vi "S7 Write.vi"(6 "Data Type":enum16{"I", "Q", "M", "D", "Count", "Timer"}(ring), 7 "DB block":u16, 8 "Error In":errorcluster, 9 "Write Byte":u8[](array[numeric]), 10 "Start Address":u16, 11 "TCP In":refnum<k5>) -> (0 "Error out":errorcluster caption="Error Out", 3 "TCP Out":refnum<k5>)   [LabVIEW 2020]
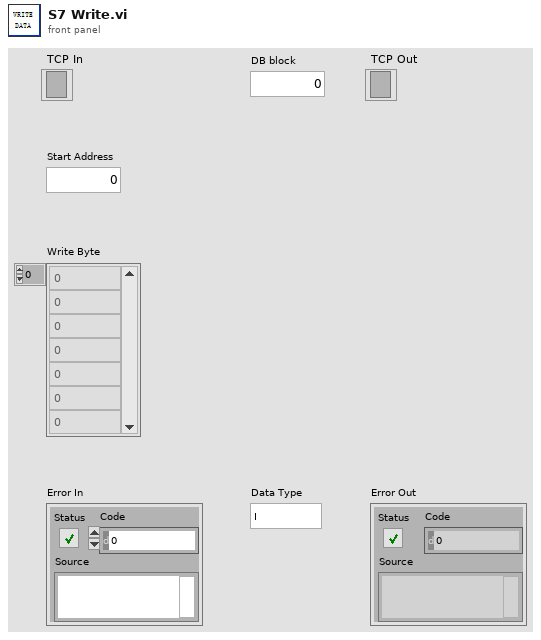
[diagram p1: front panel]
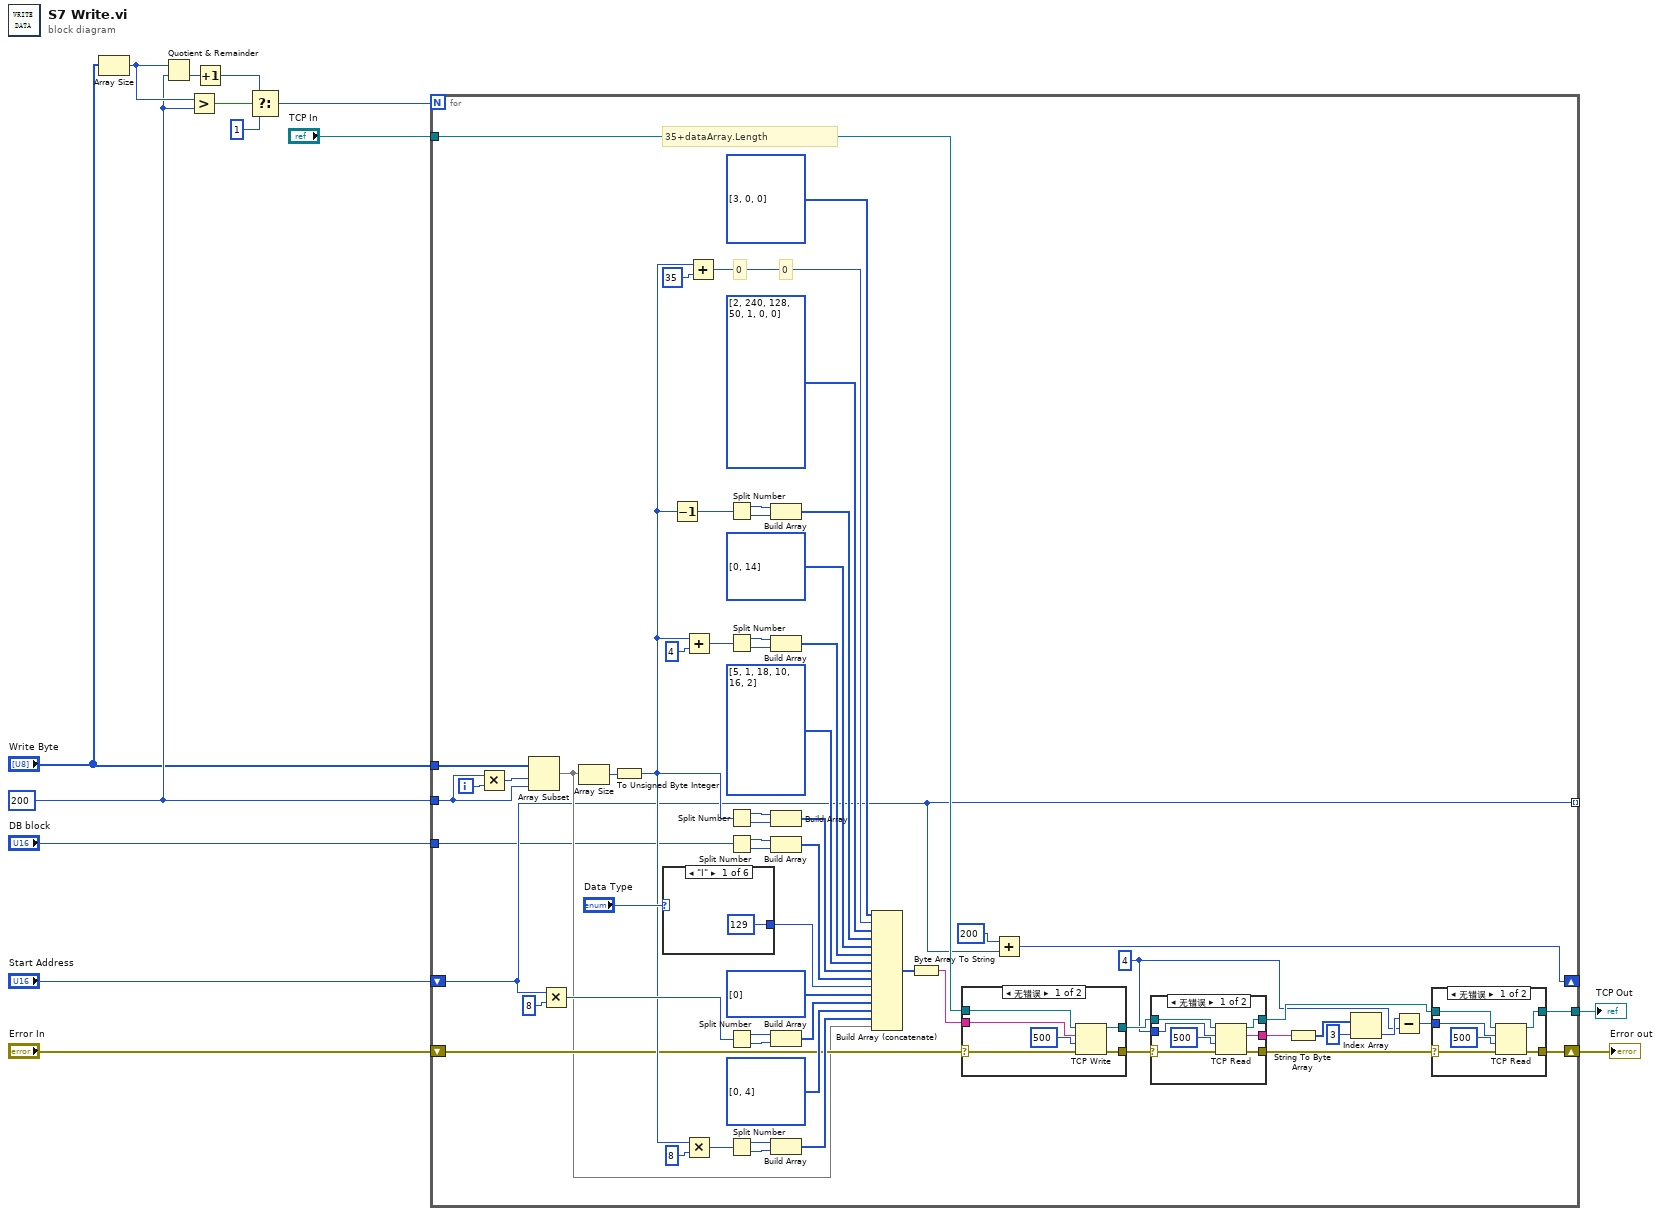
[diagram p0: block diagram]
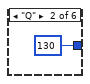
[diagram p5: hidden frame]
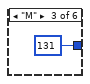
[diagram p6: hidden frame]
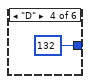
[diagram p7: hidden frame]
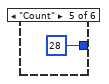
[diagram p8: hidden frame]
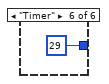
[diagram p9: hidden frame]
diagram:
  w6 = 200 ("y")
  n1 = Array Size(array="Write Byte") -> (size(s)=w7:i32)
  n2 = Quotient & Remainder(x=w7, y=w6) -> (floor(x/y)=w10:i32)  [unwired: 1 out]
  n3 = Greater?(x=w7, y=w6) -> (0:w12:bool)
  n4 = Increment(x=w10) -> (x+1=w9:i32)
  n5 = Select(t=w9, s=w12, f=1) -> (s? t:f=w8:i32)
  n6 = for {
    N: w8 -> [_]
    shift-right: [w76] -> w3
    shift-left: "Error In" -> [w28]
    tunnel: [w25] -> w14
    tunnel: "TCP In" -> [w24]
    tunnel: "Write Byte" -> [w23]
    tunnel: w6 -> [w17]
    shift-right: [w19] -> _
    shift-left: "Start Address" -> [w18]
    tunnel: [w18] -> _ mode=indexing
    tunnel: "DB block" -> [w15]
    i -> [w22]
    w33 = 4 ("超时毫秒(25000)")
    # "35+dataArray.Length"
    # "0"
    # "0"
    n7 = Multiply(x=w17, y=w22) -> (x*y=w21:i32)
    n8 = Array Subset(array=w23, index=w21, length=w17) -> (w20:u8[])
    n9 = Multiply(x=w18, y=u16 8) -> (x*y=w56:u16)
    n10 = Array Size(array=w20) -> (size(s)=w50:i32)
    n11 = To Unsigned Byte Integer(number=w50) -> (unsigned 8bit integer=w29:u8)
    n12 = case shown="\"I\"" "Data Type" {
      tunnel: [u8 129 ("DB.NO. 3") u8 130 ("DB.NO. 3") u8 131 ("DB.NO. 3") u8 132 ("DB.NO. 3") u8 28 ("DB.NO. 3") u8 29 ("DB.NO. 3")] -> w35
      frame "I" {
      }
      frame "Q" {
      }
      frame "M" {
      }
      frame "D" {
      }
      frame "Count" {
      }
      frame "Timer" {
      }
    }
    n13 = Decrement(x=w29) -> (x-1=w70:u8)
    n14 = Add(x=w29, y=u8 4) -> (x+y=w65:u8)
    n15 = Multiply(x=w29, y=u8 8) -> (x*y=w52:u8)
    n16 = Add(x=w29, y=u8 35 ("Length")) -> (x+y=w48:u8)
    n17 = Split Number(x=w70) -> (hi(x)=w69:u8, lo(x)=w68:u8)
    n18 = Split Number(x=w65) -> (hi(x)=w66:u8, lo(x)=w67:u8)
    n19 = Split Number(x=w29) -> (hi(x)=w62:u8, lo(x)=w63:u8)
    n20 = Split Number(x=w15) -> (hi(x)=w61:u8, lo(x)=w60:u8)
    n21 = Split Number(x=w56) -> (hi(x)=w58:u8, lo(x)=w57:u8)
    n22 = Split Number(x=w52) -> (hi(x)=w55:u8, lo(x)=w54:u8)
    n23 = Build Array(w69, w68) -> (w46:u8[])
    n24 = Build Array(w66, w67) -> (w44:u8[])
    n25 = Build Array(w62, w63) -> (w42:u8[])
    n26 = Build Array(w61, w60) -> (w41:u8[])
    n27 = Build Array(w58, w57) -> (w39:u8[])
    n28 = Build Array(w55, w54) -> (w30:u8[])
    n29 = Build Array (concatenate)(u8[] [3, 0, 0], w48, u8[] [2, 240, 128, 50, 1, 0, 0], w46, u8[] [0, 14], w44, u8[] [5, 1, 18, 10, 16, 2], w42, w41, w35, u8[] [0], w39, u8[] [0, 4], w30, w20) -> (w37:u8[])
    n30 = Byte Array To String(unsigned byte array=w37) -> (string=w71:string)
    n31 = case shown="无错误" w28 {
      selector: w28 -> [w94 w100]
      tunnel: [w99 w100] -> w27
      tunnel: [w98 w101] -> w72
      tunnel: w24 -> [w97 w101]
      tunnel: w71 -> [w96 _]
      frame No Error {
        n32 = TCP Write(connection ID=w97, data in=w96, error in (no error)=w94, 9:500 ("timeout ms (25000)")) -> (connection ID out=w98:refnum<k5>, error out=w99:errorcluster)  [unwired: 1 out]
      }
      frame Error {
      }
    }
    n33 = Add(x=u16 200, y=w18) -> (x+y=w19:u16)
    n34 = case shown="无错误" w27 {
      selector: w27 -> [w85 w92]
      tunnel: [w90 w92] -> w26
      tunnel: [w89 _] -> w75
      tunnel: [w88 w93] -> w73
      tunnel: w72 -> [w87 w93]
      tunnel: w33 -> [w86 _]
      frame No Error {
        n35 = TCP Read(connection ID=w87, bytes to read=w86, error in (no error)=w85, 9:500 ("读取的字节")) -> (connection ID out=w88:refnum<k5>, data out=w89:string, error out=w90:errorcluster)  [unwired: 1 in]
      }
      frame Error {
      }
    }
    n36 = String To Byte Array(string=w75) -> (unsigned byte array=w31:u8[])
    n37 = Index Array(array=w31, index=3 ("索引")) -> (element=w34:u8)
    n38 = Subtract(x=w34, y=w33) -> (x-y=w32:i32)
    n39 = case shown="无错误" w26 {
      selector: w26 -> [w77 w83]
      tunnel: [w81 w83] -> w76
      tunnel: [w80 w84] -> w25
      tunnel: w73 -> [w79 w84]
      tunnel: w32 -> [w78 _]
      frame No Error {
        n40 = TCP Read(connection ID=w79, bytes to read=w78, error in (no error)=w77, 9:500 ("读取的字节")) -> (connection ID out=w80:refnum<k5>, error out=w81:errorcluster)  [unwired: 1 in, 1 out]
      }
      frame Error {
      }
    }
  }
  "TCP Out" <- w14
  "Error out" <- w3
